vi "JSON example W7X.vi"() -> ()   [LabVIEW 2014]
uses:
  <vilib>/httpClient/LabVIEWHTTPClient.lvlib
  <vilib>/httpClient/POSTBuffer.vi
panel:
  out "GET error out":errorcluster
  out "initialized array":u64[](array[numeric])
  out "subarray":sgl[][](array[numeric])
  out "size(s)":i32[](array[numeric])
  out "JSON string 2":string
  out "sampleCount":i32
  out "label 2":string
  out "body":string
  out "values 2":dbl[][](array[numeric])
  out "dimensions 2":u64[](array[numeric])
  in  "2Dcluster":T1
  out "body 2":string
  out "headers 2":string
  out "PUT error out":errorcluster
  out "headers":string
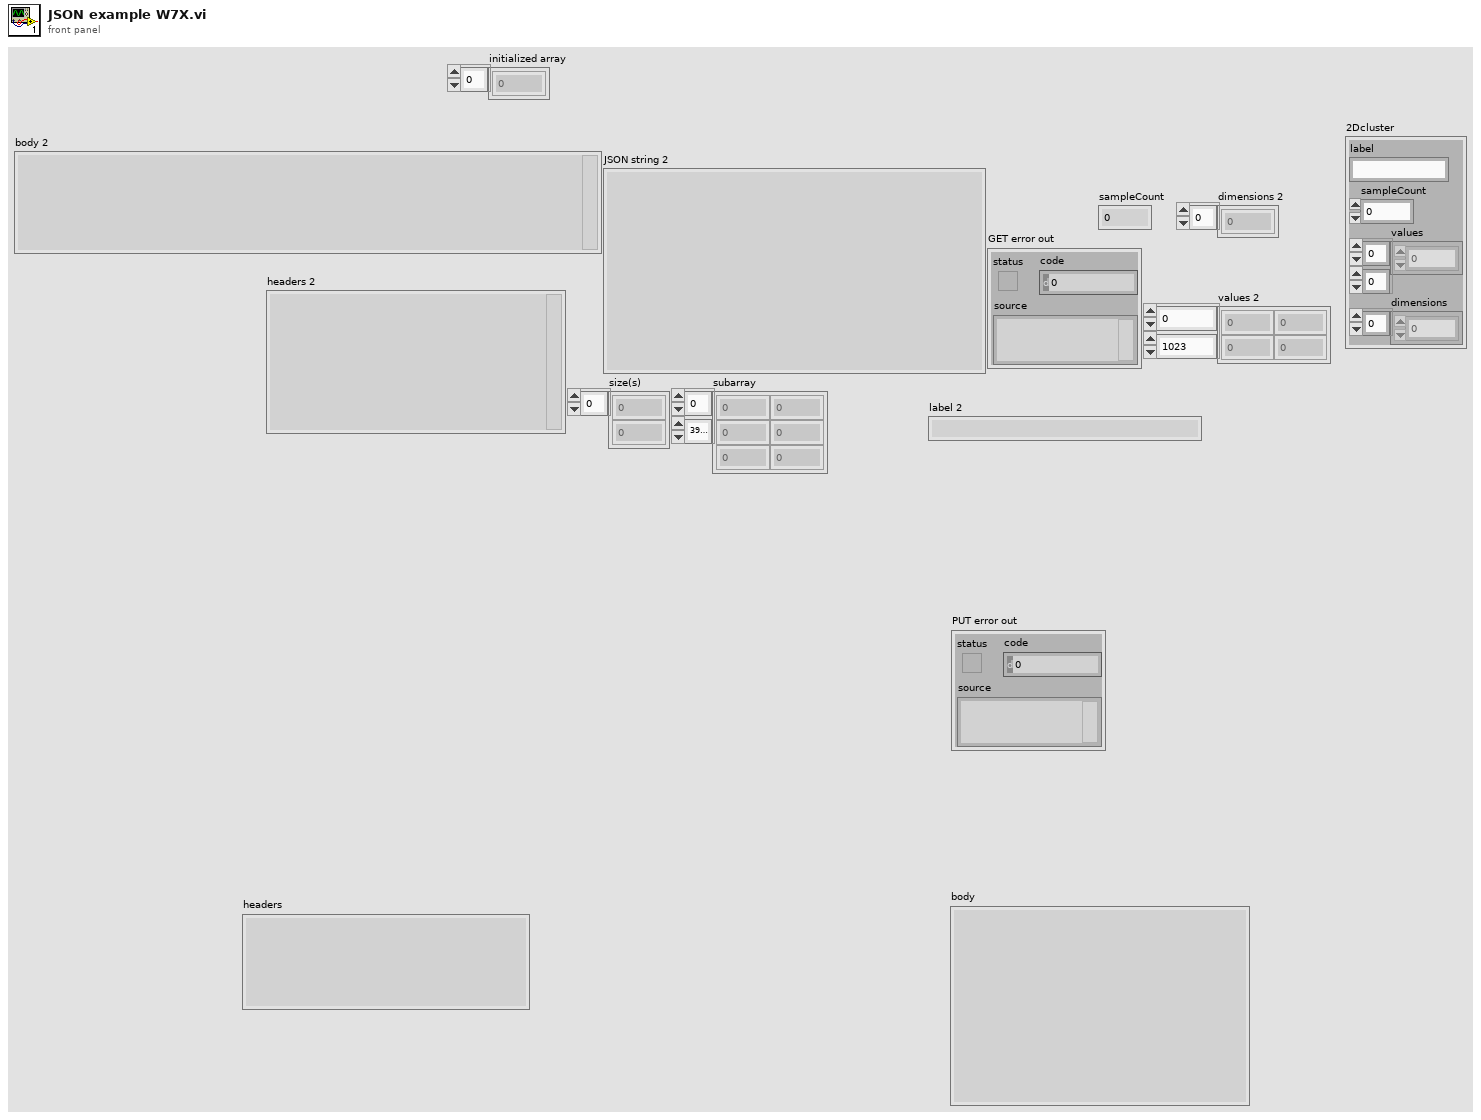
[diagram p1: front panel]
types:
  T1 = cluster{"label":string, "sampleCount":i32, "values":dbl[][], "dimensions":u64[]}
  T2 = typedef "LabVIEWHTTPClient.lvlib/ClientHandle.ctl" = refnum<k1>
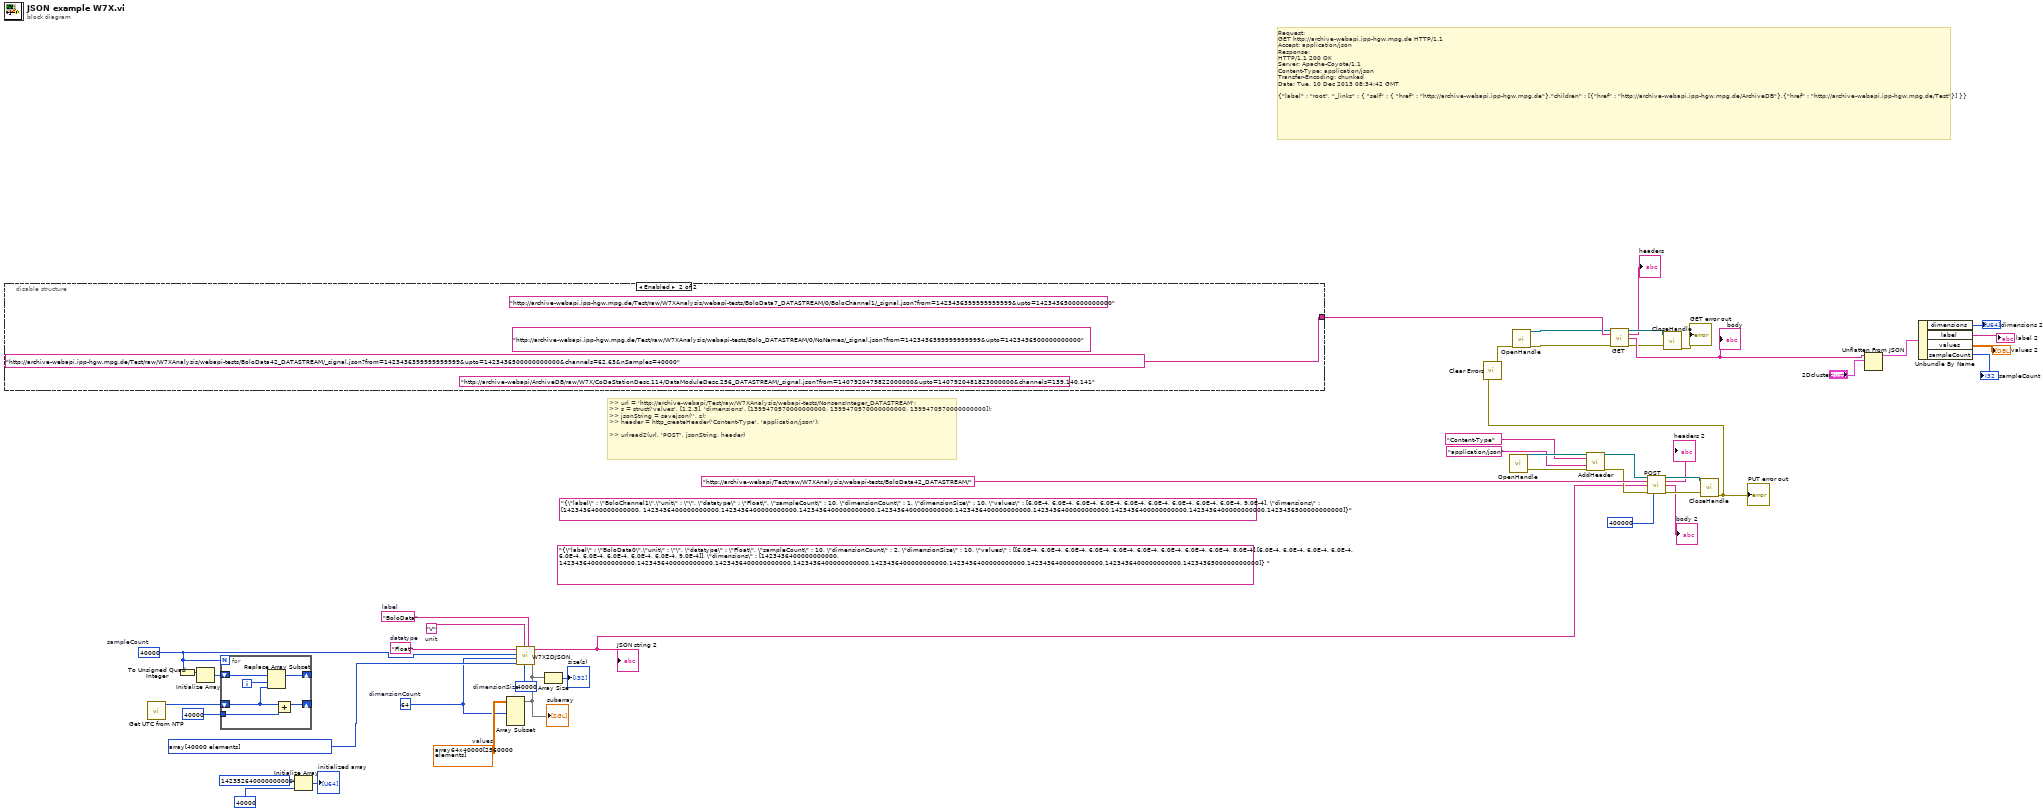
[diagram p0: block diagram]
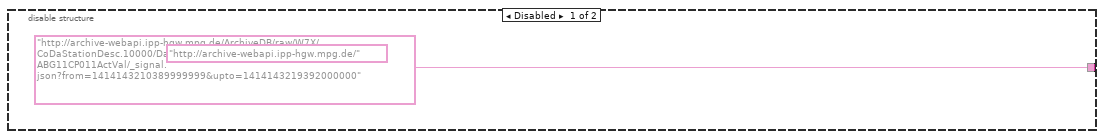
[diagram p2: hidden frame]
diagram:
  w18 = sgl[][] array64x40000[2560000 elements]  # values
  w27 = 40000  # dimensionSize
  w16 = 64  # dimensionCount
  w3 = 40000  # sampleCount
  w28 = "Float"  # datatype
  w29 = "V"  # unit
  w30 = "BoloData"  # label
  (unwired) "{\"label\" : \"BoloChannel1\",\"unit\" : \"\", \"datatype\" : \"Float\", \"sampleCount\" : 10, \"dimensionCount\" : 1, \"dimensionSize\" : 10, \"values\" : [6.0E-4, 6.0E-4, 6.0E-4, 6.0E-4, 6.0E-4, 6.0E-4, 6.0E-4, 6.0E-4, 6.0E-4, 9.0E-4], \"dimensions\" : [1423436400000000000, 1423436400000000000,1423436400000000000,1423436400000000000,1423436400000000000,1423436400000000000,1423436400000000000,1423436400000000000,1423436400000000000,1423436500000000000]}" ("String")
  (unwired) "{\"label\" : \"BoloData0\",\"unit\" : \"\", \"datatype\" : \"Float\", \"sampleCount\" : 10, \"dimensionCount\" : 2, \"dimensionSize\" : 10, \"values\" : [[6.0E-4, 6.0E-4, 6.0E-4, 6.0E-4, 6.0E-4, 6.0E-4, 6.0E-4, 6.0E-4, 6.0E-4, 8.0E-4],[6.0E-4, 6.0E-4, 6.0E-4, 6.0E-4, 6.0E-4, 6.0E-4, 6.0E-4, 6.0E-4, 6.0E-4, 9.0E-4]], \"dimensions\" : [1423436400000000000, 1423436400000000000,1423436400000000000,1423436400000000000,1423436400000000000,1423436400000000000,1423436400000000000,1423436400000000000,1423436400000000000,1423436500000000000]} " ("String")
  # "seems OK"
  # ">> url = 'http://archive-webapi/Test/raw/W7XAnalysis/webapi-tests/NonsensInteger_DATASTREAM';\n>> s = struct('values', [1,2,3], 'dimensions', [1399470570000000000, 1399470570000000000, 1399470570000000000]);\n>> jsonString = savejson('', s);\n>> header = http_createHeader('Content-Type', 'application/json');\n\n>> urlread2(url, 'POST', jsonString, header)"
  # "Request:\nGET http://archive-webapi.ipp-hgw.mpg.de HTTP/1.1\nAccept: application/json\nResponse:\nHTTP/1.1 200 OK\nServer: Apache-Coyote/1.1\nContent-Type: application/json\nTransfer-Encoding: chunked\nDate: Tue, 10 Dec 2013 08:34:42 GMT\n\n{\"label\" : \"root\", \"_links\" : { \"self\" : { \"href\" : \"http://archive-webapi.ipp-hgw.mpg.de\"},\"children\" : [{\"href\" : \"http://archive-webapi.ipp-hgw.mpg.de/ArchiveDB\"},{\"href\" : \"http://archive-webapi.ipp-hgw.mpg.de/Test\"}] }}"
  n1 = disable-structure shown="Enabled" {
    disable-tunnel: ["http://archive-webapi.ipp-hgw.mpg.de/ArchiveDB/raw/W7X/CoDaStationDesc.10000/DataModuleDesc.10006_DATASTREAM/35/ABG11CP011ActVal/_signal.json?from=1414143210389999999&upto=1414143219392000000" ("url") "http://archive-webapi.ipp-hgw.mpg.de/Test/raw/W7XAnalysis/webapi-tests/BoloData42_DATASTREAM/_signal.json?from=1423436399999999999&upto=1423436500000000000&channels=62,63&nSamples=40000" ("url")] -> w44
    frame Disabled {
      (unwired) "http://archive-webapi.ipp-hgw.mpg.de/" ("url")
    }
    frame Enabled {
      (unwired) "http://archive-webapi/ArchiveDB/raw/W7X/CoDaStationDesc.114/DataModuleDesc.256_DATASTREAM/_signal.json?from=1407920479822000000&upto=1407920481823000000&channels=139,140,141"
      (unwired) "http://archive-webapi.ipp-hgw.mpg.de/Test/raw/W7XAnalysis/webapi-tests/Bolo_DATASTREAM/0/NoNames/_signal.json?from=1423436399999999999&upto=1423436500000000000" ("url")
      (unwired) "http://archive-webapi.ipp-hgw.mpg.de/Test/raw/W7XAnalysis/webapi-tests/BoloData7_DATASTREAM/0/BoloChannel1/_signal.json?from=1423436399999999999&upto=1423436500000000000" ("url")
    }
  }
  n2 = call "Get UTC from NTP.vi"() -> ("UTC Time"=w5:i64)  [unwired: 10 in, 1 out]
  n3 = To Unsigned Quad Integer(1:w3) -> (0:w1:u64)
  n4 = Initialize Array(w1) -> (w2:u64[])  [unwired: 1 in]
  n5 = for {
    N: w3 -> [_]
    tunnel: u64 40000 ("element") -> [w49]
    shift-right: [w50] -> _
    shift-left: w5 -> [w51]
    shift-right: [w53] -> _
    shift-left: w2 -> [w54]
    i -> [w52]
    n6 = Replace Array Subset(array=w54, new element=w51, index=w52) -> (w53:u64[])
    n7 = Add(x=w51, y=w49) -> (x+y=w50:u64)
  }
  n8 = Initialize Array(u64 1423526400000000000 ("element"), 40000 ("dimension size")) -> (→"initialized array":u64[])
  n9 = Array Subset(array=w18, length (row)=w16) -> (w17:sgl[][])  [unwired: 3 in]
  "subarray" <- w17
  n10 = call "W7X2DJSON.vi"("values"=w17, "label"=w30, "dimensionSize"=w27, 7:w29, "dimensions"=u64[] array[40000 elements] ("initialized array"), "dimensionCount"=w16, "sampleCount"=w3, "datatype"=w28) -> ("JSON string"=w10:string)  [unwired: 3 in]
  "JSON string 2" <- w10
  n11 = Array Size(array=w17) -> (size(s)=→"size(s)":i32[])
  n12 = call <vilib>:"OpenHandle.vi"() -> ("client handle out"=w39:T2, "error out"=w38:errorcluster)  [unwired: 14 in]
  n13 = call <vilib>:"AddHeader.vi"("client handle"=w39, "header"="Content-Type", "value"="application/json", "error in (no error)"=w38) -> ("client handle out"=w37:T2, "error out"=w36:errorcluster)  [unwired: 10 in]
  n14 = call-poly <vilib>:"POST.vi"("client handle"=w37, "url"="http://archive-webapi/Test/raw/W7XAnalysis/webapi-tests/BoloData42_DATASTREAM/", "buffer"=w10, "error in (no error)"=w36, "timeout (10000)"=400000) -> ("client handle out"=w43:T2, "headers"=→"headers 2":string, "body"=→"body 2":string, "error out"=w42:errorcluster)  [unwired: 7 in]
  n15 = call <vilib>:"CloseHandle.vi"("client handle"=w43, "error in (no error)"=w42) -> ("error out"=w15:errorcluster)  [unwired: 13 in]
  "PUT error out" <- w15
  n16 = call <vilib>:"Clear Errors.vi"("error in (no error)"=w15) -> ("error out"=w14:errorcluster)  [unwired: 5 in, 1 out]
  n17 = call <vilib>:"OpenHandle.vi"("error in (no error)"=w14) -> ("client handle out"=w35:T2, "error out"=w34:errorcluster)  [unwired: 13 in]
  n18 = call <vilib>:"GET.vi"("client handle"=w35, "url"=w44, "error in (no error)"=w34) -> ("client handle out"=w46:T2, "headers"=→"headers":string, "body"=w23:string, "error out"=w7:errorcluster)  [unwired: 9 in]
  "body" <- w23
  n19 = call <vilib>:"CloseHandle.vi"("client handle"=w46, "error in (no error)"=w7) -> ("error out"=→"GET error out":errorcluster)  [unwired: 13 in]
  n20 = Unflatten From JSON(JSON string=w23, type and defaults="2Dcluster") -> (value=w26:T1)  [unwired: 5 in, 1 out]
  n21 = Unbundle By Name(w26) -> ("dimensions"=→"dimensions 2":u64[], "label"=→"label 2":string, "values"=→"values 2":dbl[][], "sampleCount"=→"sampleCount":i32)
